vi "HardwareRangeStrings.vi"(8 "error in (no error)":errorcluster, 11 "Pstat IN":refnum<k7>) -> (0 "error out":errorcluster, 2 "Hardware Strings":T1, 3 "Pstat OUT":refnum<k7>)   [LabVIEW 2016]
panel:
  in  "CA Speeds":string[](array[string])=["Fast\n", "Normal", "Medium", "Slow"]
  in  "Family":string="PC5"
  in  "AchFilters":string[](array[string])=["30 mV", "300 mV", "3 V", "12 V"]
  in  "IchFilters":string[](array[string])=["30 mV", "300 mV", "3 V", "12 V"]
  in  "VchFilters":string[](array[string])=["30 mV", "300 mV", "3 V", "12 V"]
  in  "AchRanges":string[](array[string])=["30 mV", "300 mV", "3 V", "12 V"]
  in  "IchRanges":string[](array[string])=["30 mV", "300 mV", "3 V", "12 V"]
  in  "VchRanges":string[](array[string])=["30 mV", "300 mV", "3 V", "12 V"]
  in  "First I/E Range":i32=1
  in  "I/E Ranges":string[](array[string])
  out "Status":i32
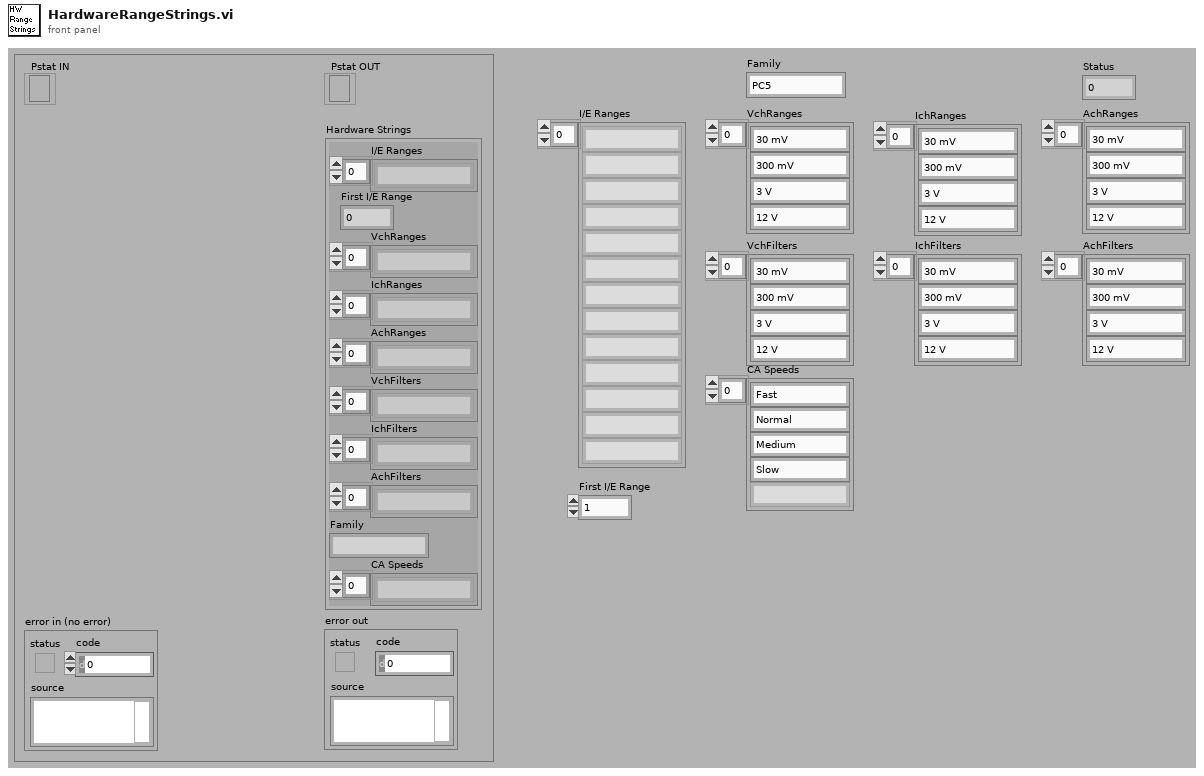
[diagram p1: front panel]
types:
  T1 = cluster{"I/E Ranges":string[], "First I/E Range":i32, "VchRanges":string[], "IchRanges":string[], "AchRanges":string[], "VchFilters":string[], "IchFilters":string[], "AchFilters":string[], "Family":string, "CA Speeds":string[]}
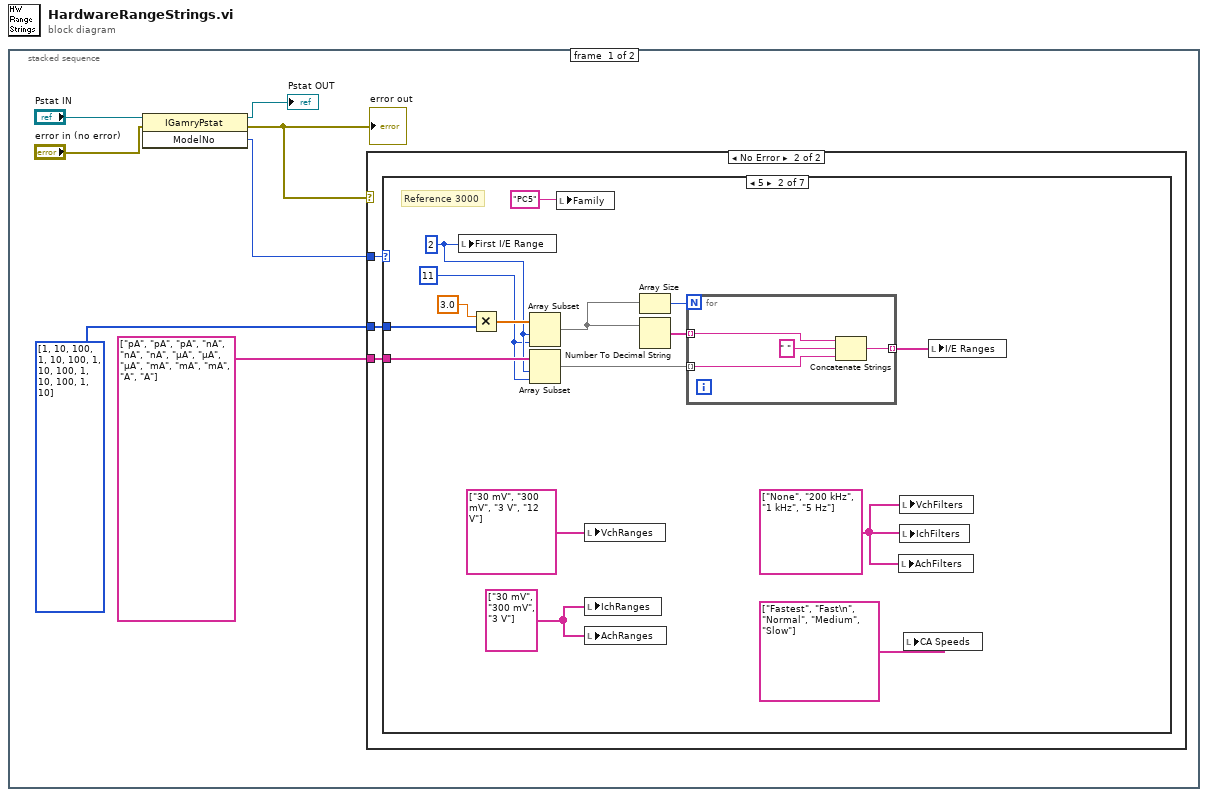
[diagram p0: block diagram]
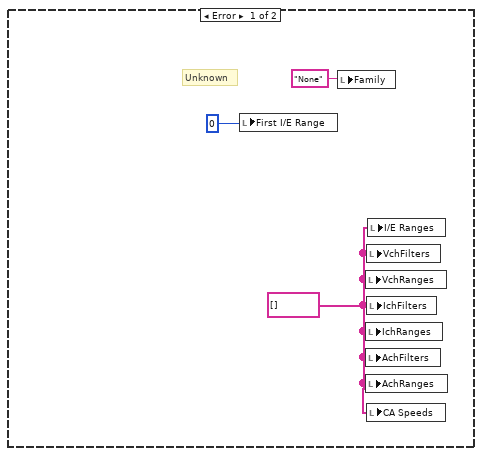
[diagram p2: hidden frame]
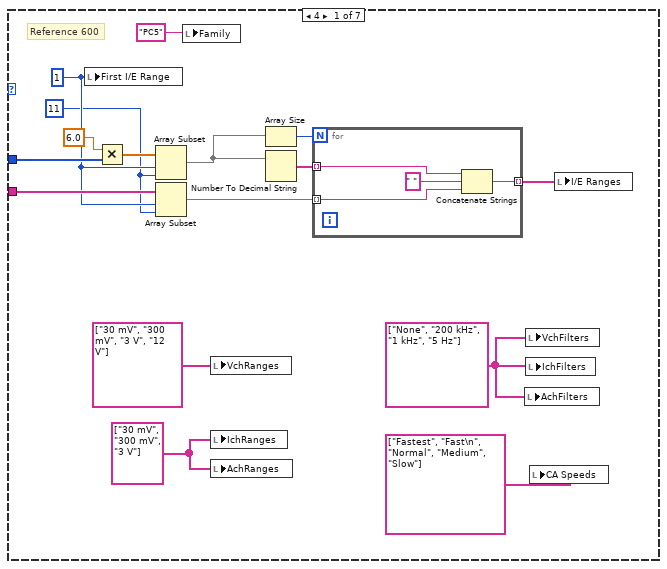
[diagram p3: hidden frame]
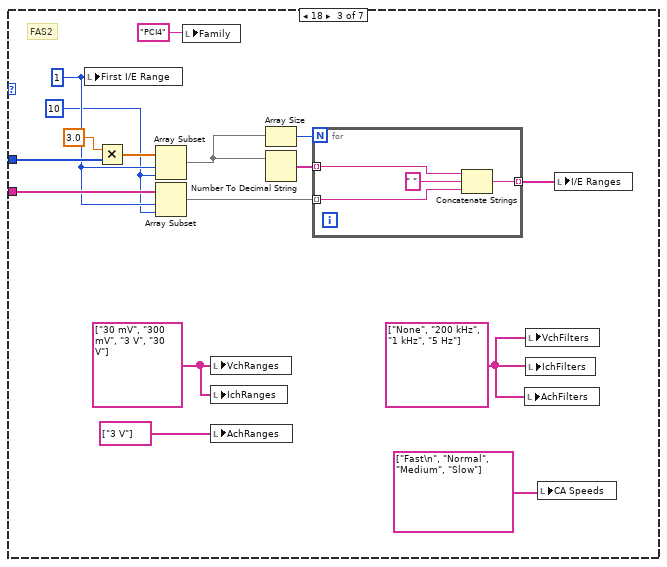
[diagram p4: hidden frame]
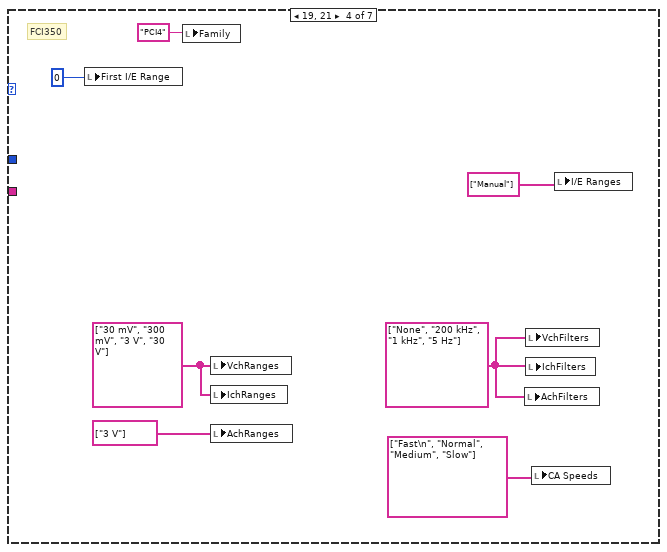
[diagram p5: hidden frame]
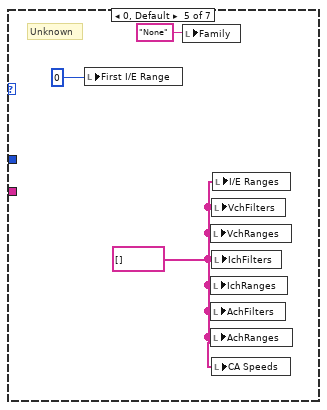
[diagram p6: hidden frame]
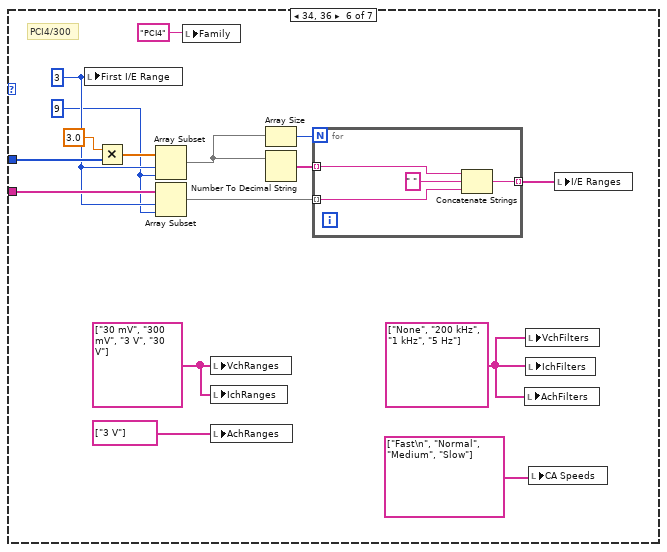
[diagram p7: hidden frame]
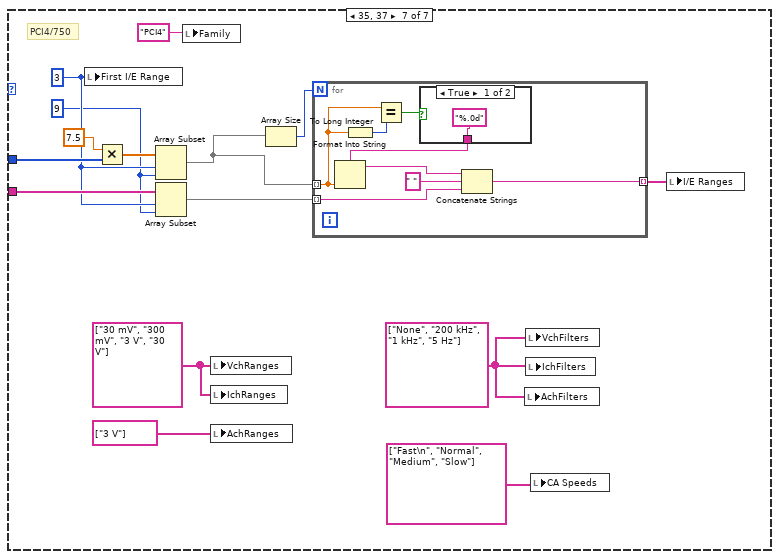
[diagram p8: hidden frame]
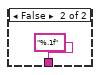
[diagram p9: hidden frame]
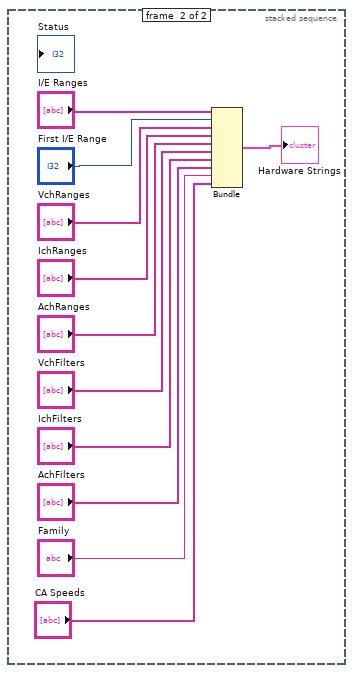
[diagram p10: hidden frame]
diagram:
  n1 = stacked-sequence {
    frame #0 {
      n2 = invoke class="IGamryPstat" method="ModelNo"(reference="Pstat IN", error in="error in (no error)") -> (reference out=→"Pstat OUT":refnum<k7>, error out=w2:errorcluster, "ModelNo"=w4:i32)  [unwired: 1 in]
      "error out" <- w2
      n3 = case shown="No Error" w2 {
        tunnel: i32[] [1, 10, 100, 1, 10, 100, 1, 10, 100, 1, 10, 100, 1, 10] -> [_ w13]
        tunnel: string[] ["pA", "pA", "pA", "nA", "nA", "nA", "µA", "µA", "µA", "mA", "mA", "mA", "A", "A"] -> [_ w12]
        tunnel: w4 -> [_ w11]
        frame Error {
          w8 = string[] []
          # "Unknown"
          n4 = local write "First I/E Range"(0) -> ()
          n5 = local write "Family"("None") -> ()
          n6 = local write "VchRanges"(w8) -> ()
          n7 = local write "IchRanges"(w8) -> ()
          n8 = local write "AchFilters"(w8) -> ()
          n9 = local write "AchRanges"(w8) -> ()
          n10 = local write "VchFilters"(w8) -> ()
          n11 = local write "IchFilters"(w8) -> ()
          n12 = local write "CA Speeds"(w8) -> ()
          n13 = local write "I/E Ranges"(w8) -> ()
        }
        frame No Error {
          n14 = case shown="5" w11 {
            tunnel: w13 -> [w25 w45 w65 _ _ w95 w114]
            tunnel: w12 -> [w27 w47 w67 _ _ w97 w116]
            frame 4 {
              w16 = string[] ["None", "200 kHz", "1 kHz", "5 Hz"]
              w17 = string[] ["30 mV", "300 mV", "3 V"]
              w20 = 1
              w19 = 11 ("length")
              # "Reference 600"
              n15 = local write "First I/E Range"(w20) -> ()
              n16 = Multiply(x=sgl 6.0, y=w25) -> (x*y=w28:sgl[])
              n17 = Array Subset(array=w28, index=w20, length=w19) -> (w24:sgl[])
              n18 = Array Subset(array=w27, index=w20, length=w19) -> (w23:string[])
              n19 = local write "Family"("PC5") -> ()
              n20 = local write "VchRanges"(string[] ["30 mV", "300 mV", "3 V", "12 V"]) -> ()
              n21 = local write "IchRanges"(w17) -> ()
              n22 = local write "AchRanges"(w17) -> ()
              n23 = Array Size(array=w24) -> (size(s)=w26:i32)
              n24 = Number To Decimal String(number=w24) -> (decimal integer string=w22:string[])  [unwired: 1 in]
              n25 = for {
                N: w26 -> [_]
                tunnel: w23 -> [w32] mode=indexing
                tunnel: w22 -> [w31] mode=indexing
                tunnel: [w30] -> w21 mode=indexing
                n26 = Concatenate Strings(w31, " " ("string"), w32) -> (w30:string)
              }
              n27 = local write "AchFilters"(w16) -> ()
              n28 = local write "VchFilters"(w16) -> ()
              n29 = local write "IchFilters"(w16) -> ()
              n30 = local write "CA Speeds"(string[] ["Fastest", "Fast\n", "Normal", "Medium", "Slow"]) -> ()
              n31 = local write "I/E Ranges"(w21) -> ()
            }
            frame 5 {
              w36 = string[] ["None", "200 kHz", "1 kHz", "5 Hz"]
              w37 = string[] ["30 mV", "300 mV", "3 V"]
              w40 = 2
              w39 = 11 ("length")
              # "Reference 3000"
              n32 = local write "First I/E Range"(w40) -> ()
              n33 = Multiply(x=sgl 3.0, y=w45) -> (x*y=w48:sgl[])
              n34 = Array Subset(array=w48, index=w40, length=w39) -> (w44:sgl[])
              n35 = Array Subset(array=w47, index=w40, length=w39) -> (w43:string[])
              n36 = local write "Family"("PC5") -> ()
              n37 = local write "VchRanges"(string[] ["30 mV", "300 mV", "3 V", "12 V"]) -> ()
              n38 = local write "IchRanges"(w37) -> ()
              n39 = local write "AchRanges"(w37) -> ()
              n40 = Array Size(array=w44) -> (size(s)=w46:i32)
              n41 = Number To Decimal String(number=w44) -> (decimal integer string=w42:string[])  [unwired: 1 in]
              n42 = for {
                N: w46 -> [_]
                tunnel: w43 -> [w52] mode=indexing
                tunnel: w42 -> [w51] mode=indexing
                tunnel: [w50] -> w41 mode=indexing
                n43 = Concatenate Strings(w51, " " ("string"), w52) -> (w50:string)
              }
              n44 = local write "AchFilters"(w36) -> ()
              n45 = local write "VchFilters"(w36) -> ()
              n46 = local write "IchFilters"(w36) -> ()
              n47 = local write "CA Speeds"(string[] ["Fastest", "Fast\n", "Normal", "Medium", "Slow"]) -> ()
              n48 = local write "I/E Ranges"(w41) -> ()
            }
            frame 18 {
              w58 = string[] ["None", "200 kHz", "1 kHz", "5 Hz"]
              w56 = string[] ["30 mV", "300 mV", "3 V", "30 V"]
              w60 = 1
              w59 = 10 ("length")
              # "FAS2"
              n49 = local write "First I/E Range"(w60) -> ()
              n50 = Multiply(x=sgl 3.0, y=w65) -> (x*y=w68:sgl[])
              n51 = Array Subset(array=w68, index=w60, length=w59) -> (w64:sgl[])
              n52 = Array Subset(array=w67, index=w60, length=w59) -> (w63:string[])
              n53 = local write "Family"("PCI4") -> ()
              n54 = local write "VchRanges"(w56) -> ()
              n55 = local write "IchRanges"(w56) -> ()
              n56 = local write "AchRanges"(string[] ["3 V"]) -> ()
              n57 = Array Size(array=w64) -> (size(s)=w66:i32)
              n58 = Number To Decimal String(number=w64) -> (decimal integer string=w62:string[])  [unwired: 1 in]
              n59 = for {
                N: w66 -> [_]
                tunnel: w63 -> [w72] mode=indexing
                tunnel: w62 -> [w71] mode=indexing
                tunnel: [w70] -> w61 mode=indexing
                n60 = Concatenate Strings(w71, " " ("string"), w72) -> (w70:string)
              }
              n61 = local write "AchFilters"(w58) -> ()
              n62 = local write "VchFilters"(w58) -> ()
              n63 = local write "IchFilters"(w58) -> ()
              n64 = local write "CA Speeds"(string[] ["Fast\n", "Normal", "Medium", "Slow"]) -> ()
              n65 = local write "I/E Ranges"(w61) -> ()
            }
            frame 19, 21 {
              w79 = string[] ["None", "200 kHz", "1 kHz", "5 Hz"]
              w77 = string[] ["30 mV", "300 mV", "3 V", "30 V"]
              # "FCI350"
              n66 = local write "First I/E Range"(0) -> ()
              n67 = local write "Family"("PCI4") -> ()
              n68 = local write "VchRanges"(w77) -> ()
              n69 = local write "IchRanges"(w77) -> ()
              n70 = local write "AchRanges"(string[] ["3 V"]) -> ()
              n71 = local write "AchFilters"(w79) -> ()
              n72 = local write "VchFilters"(w79) -> ()
              n73 = local write "IchFilters"(w79) -> ()
              n74 = local write "CA Speeds"(string[] ["Fast\n", "Normal", "Medium", "Slow"]) -> ()
              n75 = local write "I/E Ranges"(string[] ["Manual"]) -> ()
            }
            frame 0, Default {
              w81 = string[] []
              # "Unknown"
              n76 = local write "First I/E Range"(0) -> ()
              n77 = local write "Family"("None") -> ()
              n78 = local write "VchRanges"(w81) -> ()
              n79 = local write "IchRanges"(w81) -> ()
              n80 = local write "AchFilters"(w81) -> ()
              n81 = local write "AchRanges"(w81) -> ()
              n82 = local write "VchFilters"(w81) -> ()
              n83 = local write "IchFilters"(w81) -> ()
              n84 = local write "CA Speeds"(w81) -> ()
              n85 = local write "I/E Ranges"(w81) -> ()
            }
            frame 34, 36 {
              w88 = string[] ["None", "200 kHz", "1 kHz", "5 Hz"]
              w86 = string[] ["30 mV", "300 mV", "3 V", "30 V"]
              w90 = 3
              w89 = 9 ("length")
              # "PCI4/300"
              n86 = local write "First I/E Range"(w90) -> ()
              n87 = Multiply(x=sgl 3.0, y=w95) -> (x*y=w98:sgl[])
              n88 = Array Subset(array=w98, index=w90, length=w89) -> (w94:sgl[])
              n89 = Array Subset(array=w97, index=w90, length=w89) -> (w93:string[])
              n90 = local write "Family"("PCI4") -> ()
              n91 = local write "VchRanges"(w86) -> ()
              n92 = local write "IchRanges"(w86) -> ()
              n93 = local write "AchRanges"(string[] ["3 V"]) -> ()
              n94 = Array Size(array=w94) -> (size(s)=w96:i32)
              n95 = Number To Decimal String(number=w94) -> (decimal integer string=w92:string[])  [unwired: 1 in]
              n96 = for {
                N: w96 -> [_]
                tunnel: w93 -> [w102] mode=indexing
                tunnel: w92 -> [w101] mode=indexing
                tunnel: [w100] -> w91 mode=indexing
                n97 = Concatenate Strings(w101, " " ("string"), w102) -> (w100:string)
              }
              n98 = local write "AchFilters"(w88) -> ()
              n99 = local write "VchFilters"(w88) -> ()
              n100 = local write "IchFilters"(w88) -> ()
              n101 = local write "CA Speeds"(string[] ["Fast\n", "Normal", "Medium", "Slow"]) -> ()
              n102 = local write "I/E Ranges"(w91) -> ()
            }
            frame 35, 37 {
              w109 = string[] ["None", "200 kHz", "1 kHz", "5 Hz"]
              w107 = string[] ["30 mV", "300 mV", "3 V", "30 V"]
              w111 = 3
              w110 = 9 ("length")
              # "PCI4/750"
              n103 = local write "First I/E Range"(w111) -> ()
              n104 = Multiply(x=sgl 7.5, y=w114) -> (x*y=w117:sgl[])
              n105 = Array Subset(array=w117, index=w111, length=w110) -> (w105:sgl[])
              n106 = Array Subset(array=w116, index=w111, length=w110) -> (w113:string[])
              n107 = local write "Family"("PCI4") -> ()
              n108 = local write "VchRanges"(w107) -> ()
              n109 = local write "IchRanges"(w107) -> ()
              n110 = local write "AchRanges"(string[] ["3 V"]) -> ()
              n111 = Array Size(array=w105) -> (size(s)=w115:i32)
              n112 = for {
                N: w115 -> [_]
                tunnel: w113 -> [w125] mode=indexing
                tunnel: [w124] -> w112 mode=indexing
                tunnel: w105 -> [w121] mode=indexing
                n113 = To Long Integer(number=w121) -> (32bit integer=w122:i32)
                n114 = Equal?(x=w121, y=w122) -> (x = y?=w120:bool)
                n115 = case shown="True" w120 {
                  tunnel: ["%.0d" ("format string") "%.1f" ("format string")] -> w119
                  frame True {
                  }
                  frame False {
                  }
                }
                n116 = Format Into String(format string=w119, w121) -> (resulting string=w123:string)  [unwired: 2 in, 1 out]
                n117 = Concatenate Strings(w123, " " ("string"), w125) -> (w124:string)
              }
              n118 = local write "AchFilters"(w109) -> ()
              n119 = local write "VchFilters"(w109) -> ()
              n120 = local write "IchFilters"(w109) -> ()
              n121 = local write "CA Speeds"(string[] ["Fast\n", "Normal", "Medium", "Slow"]) -> ()
              n122 = local write "I/E Ranges"(w112) -> ()
            }
          }
        }
      }
    }
    frame #1 {
      n123 = Bundle("I/E Ranges"="I/E Ranges", "First I/E Range"="First I/E Range", "VchRanges"="VchRanges", "IchRanges"="IchRanges", "AchRanges"="AchRanges", "VchFilters"="VchFilters", "IchFilters"="IchFilters", "AchFilters"="AchFilters", "Family"="Family", "CA Speeds"="CA Speeds") -> (→"Hardware Strings":T1)  [unwired: 1 in]
    }
  }
